vi "ChangePBTime.vi"(7 "Instruction to change":i32, 8 "Time":dbl, 9 "Cluster":T18 {"Red MOT 88 Inputs"."Phase Times" format="%.0p"; "Red MOT 87 Inputs"."Phase Times" format="%.0p"; "ODT Params"."Phase Times (s)" format="%#_6p"; "SR400 Settings"."Port 2 Mode" items=["Scan"=1, "Fixed"=0]; "SR400 Settings"."Port 2 Scan Increment" min=-0.5 max=0.5; "SR400 Settings"."Port 2 Voltage" min=-10.0 max=10.0; "SR400 Settings"."Port 1 Scan Increment" min=-0.5 max=-0.5; "SR400 Settings"."Port 1 Voltage" min=-10.0 max=10.0; "SR400 Settings"."Port 1 Mode" items=["Scan"=1, "Fixed"=0]; "SR400 Settings"."Dwell Time (s)" min=0.002 max=60.0 format="%#_6p"; "SR400 Settings"."N Periods" min=1.0 max=2000.0 step=1.0; "SR400 Settings"."Channel T"."Trigger Preset" min=1.0 max=900000000000.0 format="%#_1e"; "SR400 Settings"."Channel T"."T Discriminator Level (V)" min=-0.3 max=0.3 format="%#_6p"; "SR400 Settings"."Channel T"."Trigger Level (V)" min=-2.0 max=2.0 format="%#_6p"; "SR400 Settings"."Channel T"."Input" items=["10 MHz", "Input 2", "Trig"]; "SR400 Settings"."Channel B"."Scan Increment (s)" min=0.0 max=0.09992 format="%#_6p"; "SR400 Settings"."Channel B"."B Gate Width (s)" min=5e-09 max=0.9992 format="%#_6p"; "SR400 Settings"."Channel B"."B Gate Delay (s)" min=0.0 max=0.9992 format="%#_6p"; "SR400 Settings"."Channel B"."B Discriminator Level (V)" min=-0.3 max=0.3 format="%#_6p"; "SR400 Settings"."Channel B"."Input" items=["Input 2"=2, "Input 1"=1]; "SR400 Settings"."Channel A"."Scan Increment (s)" min=0.0 max=0.09992 format="%#_6p"; "SR400 Settings"."Channel A"."A Gate Width (s)" min=5e-09 max=0.9992 format="%#_6p"; "SR400 Settings"."Channel A"."A Gate Delay (s)" min=0.0 max=0.9992 format="%#_6p"; "SR400 Settings"."Channel A"."A Discriminator Level (V)" min=-0.3 max=0.3 format="%#_6p"; "SR400 Settings"."Channel A"."Input" items=["Input 1", "10 MHz"]}) -> (1 "Time out":dbl, 2 "Cluster 2":T18 {"Red MOT 88 Inputs"."Phase Times" format="%.0p"; "Red MOT 87 Inputs"."Phase Times" format="%.0p"; "ODT Params"."Phase Times (s)" format="%#_6p"; "SR400 Settings"."Port 2 Mode" items=["Scan"=1, "Fixed"=0]; "SR400 Settings"."Port 2 Scan Increment" min=-0.5 max=0.5; "SR400 Settings"."Port 2 Voltage" min=-10.0 max=10.0; "SR400 Settings"."Port 1 Scan Increment" min=-0.5 max=-0.5; "SR400 Settings"."Port 1 Voltage" min=-10.0 max=10.0; "SR400 Settings"."Port 1 Mode" items=["Scan"=1, "Fixed"=0]; "SR400 Settings"."Dwell Time (s)" min=0.002 max=60.0 format="%#_6p"; "SR400 Settings"."N Periods" min=1.0 max=2000.0 step=1.0; "SR400 Settings"."Channel T"."Trigger Preset" min=1.0 max=900000000000.0 format="%#_1e"; "SR400 Settings"."Channel T"."T Discriminator Level (V)" min=-0.3 max=0.3 format="%#_6p"; "SR400 Settings"."Channel T"."Trigger Level (V)" min=-2.0 max=2.0 format="%#_6p"; "SR400 Settings"."Channel T"."Input" items=["10 MHz", "Input 2", "Trig"]; "SR400 Settings"."Channel B"."Scan Increment (s)" min=0.0 max=0.09992 format="%#_6p"; "SR400 Settings"."Channel B"."B Gate Width (s)" min=5e-09 max=0.9992 format="%#_6p"; "SR400 Settings"."Channel B"."B Gate Delay (s)" min=0.0 max=0.9992 format="%#_6p"; "SR400 Settings"."Channel B"."B Discriminator Level (V)" min=-0.3 max=0.3 format="%#_6p"; "SR400 Settings"."Channel B"."Input" items=["Input 2"=2, "Input 1"=1]; "SR400 Settings"."Channel A"."Scan Increment (s)" min=0.0 max=0.09992 format="%#_6p"; "SR400 Settings"."Channel A"."A Gate Width (s)" min=5e-09 max=0.9992 format="%#_6p"; "SR400 Settings"."Channel A"."A Gate Delay (s)" min=0.0 max=0.9992 format="%#_6p"; "SR400 Settings"."Channel A"."A Discriminator Level (V)" min=-0.3 max=0.3 format="%#_6p"; "SR400 Settings"."Channel A"."Input" items=["Input 1", "10 MHz"]})   [LabVIEW 2013]
uses:
  6733_Red_MOT/6733_control_panel.ctl
  6733_Red_MOT/6733_waveform_parameter_array.ctl
  6733_Red_MOT/6733_waveform_item.ctl
  6733_Red_MOT/6733_voltage_conversions.ctl
  Controls/6704/6704_static_voltages_control.ctl
  Controls/6704/static_voltage_conversions.ctl
  6221 arb waveforms/6221_panel.ctl
  6221 arb waveforms/6221_waveform_param.ctl
  Controls/SR400/SR400.ctl
  Controls/SR400/Channel A/channelA.ctl
  Controls/SR400/Channel A/channelA_inputs.ctl
  Controls/SR400/discrim_slope.ctl
  Controls/SR400/gate_mode.ctl
  Controls/SR400/Channel B/channelB.ctl
  Controls/SR400/Channel B/inputsB.ctl
  Controls/SR400/Channel T/channelT.ctl
  Controls/SR400/Channel T/inputsT.ctl
panel:
  # "(0) 689 Center Freq"
  # "(1) 689 Dither Amp"
  # "(2) 689 Power Lock"
  # "(3) Red MOT Field Grad"
  # "(0) 689 Center Freq"
  # "(1) 689 Dither Amp"
  # "(2) 689 Power Lock"
  # "(3) Red MOT Field Grad"
  # "(0) 689 Center Freq"
  # "(1) 689 Dither Amp"
  # "(2) 689 Power Lock"
  # "(3) Red MOT Field Grad"
  # "(0) 689 Center Freq"
  # "(1) 689 Dither Amp"
  # "(2) 689 Power Lock"
  # "(3) Red MOT Field Grad"
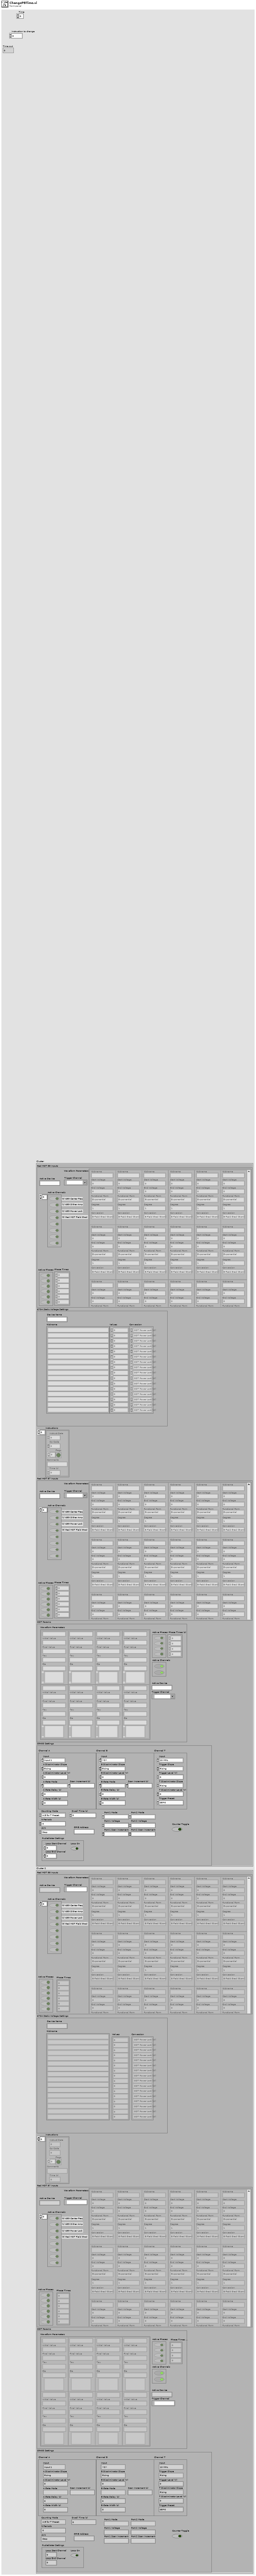
[diagram p1: front panel]
types:
  T1 = typedef "6733_control_panel.ctl" = cluster{"Active Device":string, "Active Channels":bool[], "Waveform Parameters":T2, "Active Phases":bool[], "Phase Times":dbl[], "Trigger Channel":tag}
  T2 = typedef "6733_waveform_parameter_array.ctl" = T3[][]
  T3 = typedef "6733_waveform_item.ctl" = cluster{"Functional Form":enum16{"Polynomial", "Exponential"}, "Start Voltage":dbl, "End Voltage":dbl, "Degree":i8, "Nickname":string, "Conversion":T4}
  T4 = typedef "6733_voltage_conversions.ctl" = enum16{"B Field Grad (G/cm)", "Red AOM Center Freq (MHz)", "Red Dither Pk(kHz)", "Red Power (mW)", "Volts"}
  T5 = typedef "6704_static_voltages_control.ctl" = cluster{"Device Name":string, "Values":dbl[], "Nickname":string[], "Conversion":T6[]}
  T6 = typedef "static_voltage_conversions.ctl" = enum16{"Volts", "ODT Power Lock (W)", "Sat Abs Detuning (MHz)", "Blue Mot Power Lock (mW)"}
  T7 = typedef "6221_panel.ctl" = cluster{"Waveform Parameters":T8[][], "Active Phases":bool[], "Active Channels":bool[], "Phase Times (s)":dbl[], "Active Device":string, "Trigger Channel":tag}
  T8 = typedef "6221_waveform_param.ctl" = cluster{"Initial Value":dbl, "Final Value":dbl, "Tau":dbl, "Eta":dbl, "Nickname":string, "Enum":enum16{"Volts to Volts", "Power Law", "Evaporation Formula"}}
  T9 = typedef "SR400.ctl" = cluster{"Channel A":T10, "Channel B":T14, "Channel T":T16, "N Periods":dbl, "At N":enum16{"Stop", "Start"}, "Counting Mode":enum16{"A,B for T Preset", "A-B for T Preset", "A+B for T Preset"}, "GPIB Address":string, "Dwell Time (s)":dbl, "Port 1 Mode":i32, "Port 1 Voltage":dbl, "Port 1 Scan Increment":dbl, "Port 2 Voltage":dbl, "Port 2 Scan Increment":dbl, "Port 2 Mode":i32, "Counter Toggle":bool, "Pusleblater Settings":cluster{"Loop Start Channel":dbl, "Loop End Channel":dbl, "Loop On":bool}}
  T10 = typedef "channelA.ctl" = cluster{"Input":T11, "A Discriminator Level (V)":dbl, "A Discriminator Slope":T12, "A Gate Mode":T13, "A Gate Delay (s)":dbl, "A Gate Width (s)":dbl, "Scan Increment (s)":dbl}
  T11 = typedef "channelA_inputs.ctl" = u16
  T12 = typedef "discrim_slope.ctl" = enum16{"Rising", "Falling"}
  T13 = typedef "gate_mode.ctl" = enum16{"CW", "Fixed", "Scan"}
  T14 = typedef "channelB.ctl" = cluster{"Input":T15, "B Discriminator Level (V)":dbl, "B Discriminator Slope":T12, "B Gate Mode":T13, "B Gate Delay (s)":dbl, "B Gate Width (s)":dbl, "Scan Increment (s)":dbl}
  T15 = typedef "inputsB.ctl" = u16
  T16 = typedef "channelT.ctl" = cluster{"Input":T17, "Trigger Level (V)":dbl, "Trigger Slope":T12, "T Discriminator Slope":T12, "T Discriminator Level (V)":dbl, "Trigger Preset":dbl}
  T17 = typedef "inputsT.ctl" = u16
  T18 = cluster{"Red MOT 88 Inputs":T1, "6704 Static Voltage Settings":T5, "Instructions":cluster{"Instruct Data":i32, "Op Code":i32, "Flags":bool[], "Comments":string, "Time (s)":dbl}[], "Red MOT 87 Inputs":T1, "ODT Params":T7, "SR400 Settings":T9}
  T19 = cluster{"Instruct Data":i32, "Op Code":i32, "Flags":bool[], "Comments":string, "Time (s)":dbl}[]
  T20 = cluster{"Instruct Data":i32, "Op Code":i32, "Flags":bool[], "Comments":string, "Time (s)":dbl}
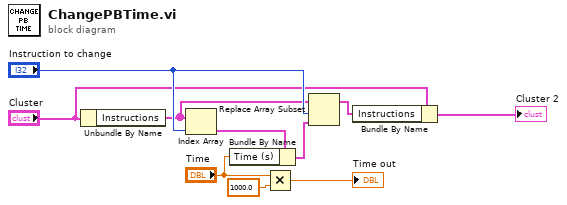
[diagram p0: block diagram]
diagram:
  n1 = Unbundle By Name("Cluster") -> ("Instructions"=w4:T19)
  n2 = Index Array(array=w4, index="Instruction to change") -> (element=w8:T20)
  n3 = Bundle By Name(cluster=w8, "Time (s)"="Time") -> (w6:T20)
  n4 = Multiply(x="Time", y=1000.0) -> (x*y=→"Time out":dbl)
  n5 = Replace Array Subset(array=w4, new element=w6, index="Instruction to change") -> (w3:T19)
  n6 = Bundle By Name(cluster="Cluster", "Instructions"=w3) -> (→"Cluster 2":T18)
